vi "Actor Core.vi"(8 "error in":errorcluster, 11 "Alpha UI in":refnum<class "Simulated Entry Console.lvclass">) -> (0 "error out":errorcluster, 3 "Actor out":refnum<class "Actor.lvclass">)   [LabVIEW 2012, in "Simulated Entry Console.lvlib" / "Simulated Entry Console.lvclass"]
doc: "(<B>Filename</B>: Actor Framework.lvlib:Actor.lvclass:Actor Core.vi)\n\nReceives messages to the actor, reacts to them, and initiates any error handling that may shut the actor down.\n\nDescendant classes may override this VI to append parallel tasks for the actor to complete while it handles messages. Overrides use the Call Parent Method node."
uses:
  Simulated Entry Console.lvclass
  <vilib>/ActorFramework/Actor/Actor.lvclass
  <vilib>/ActorFramework/Stop Msg/Stop Msg.lvclass
  Entry Console API/Entry Console API/Entry Console API.lvclass
  Car Wash Controller/Car Wash Controller/Car Wash Controller.lvclass
  Car Wash Controller/Car Wash Controller/Wash Step.ctl
panel:
  in  "Start":bool
  in  "Button 8":bool
  in  "Button 7":bool
  in  "Button 6":bool
  in  "Button 5":bool
  in  "Button 4":bool
  in  "Button 3":bool
  in  "Button 2":bool
  in  "Under Body Wash":bool
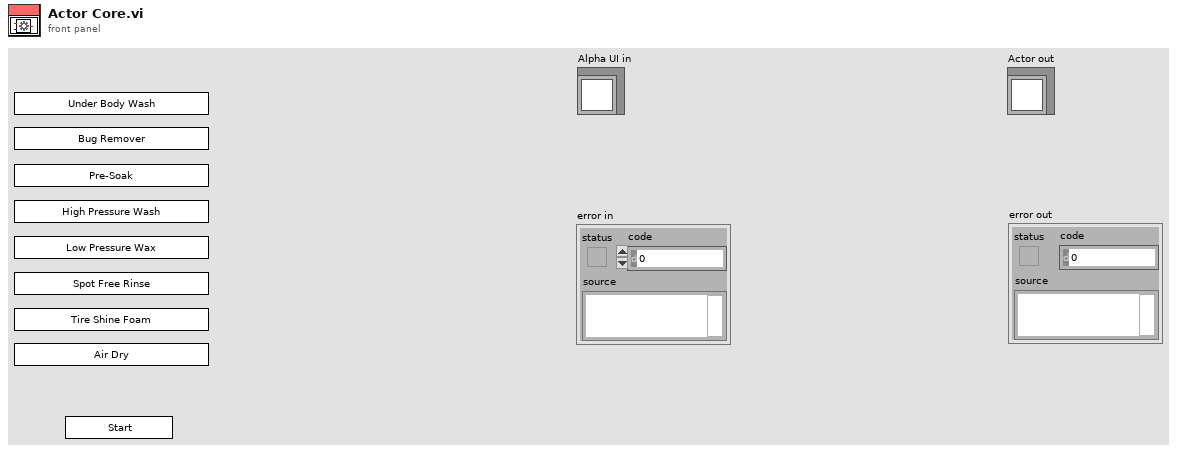
[diagram p1: front panel]
types:
  T1 = typedef "Car Wash Controller.lvlib/Car Wash Controller.lvclass/Wash Step.ctl" = enum16{"Under Body Wash", "Bug Remover", "Pre-Soak", "High Pressure Wash", "Low Pressure Wax", "Spot Free Rince", "Tire Shine Foam", "Air Dry"}
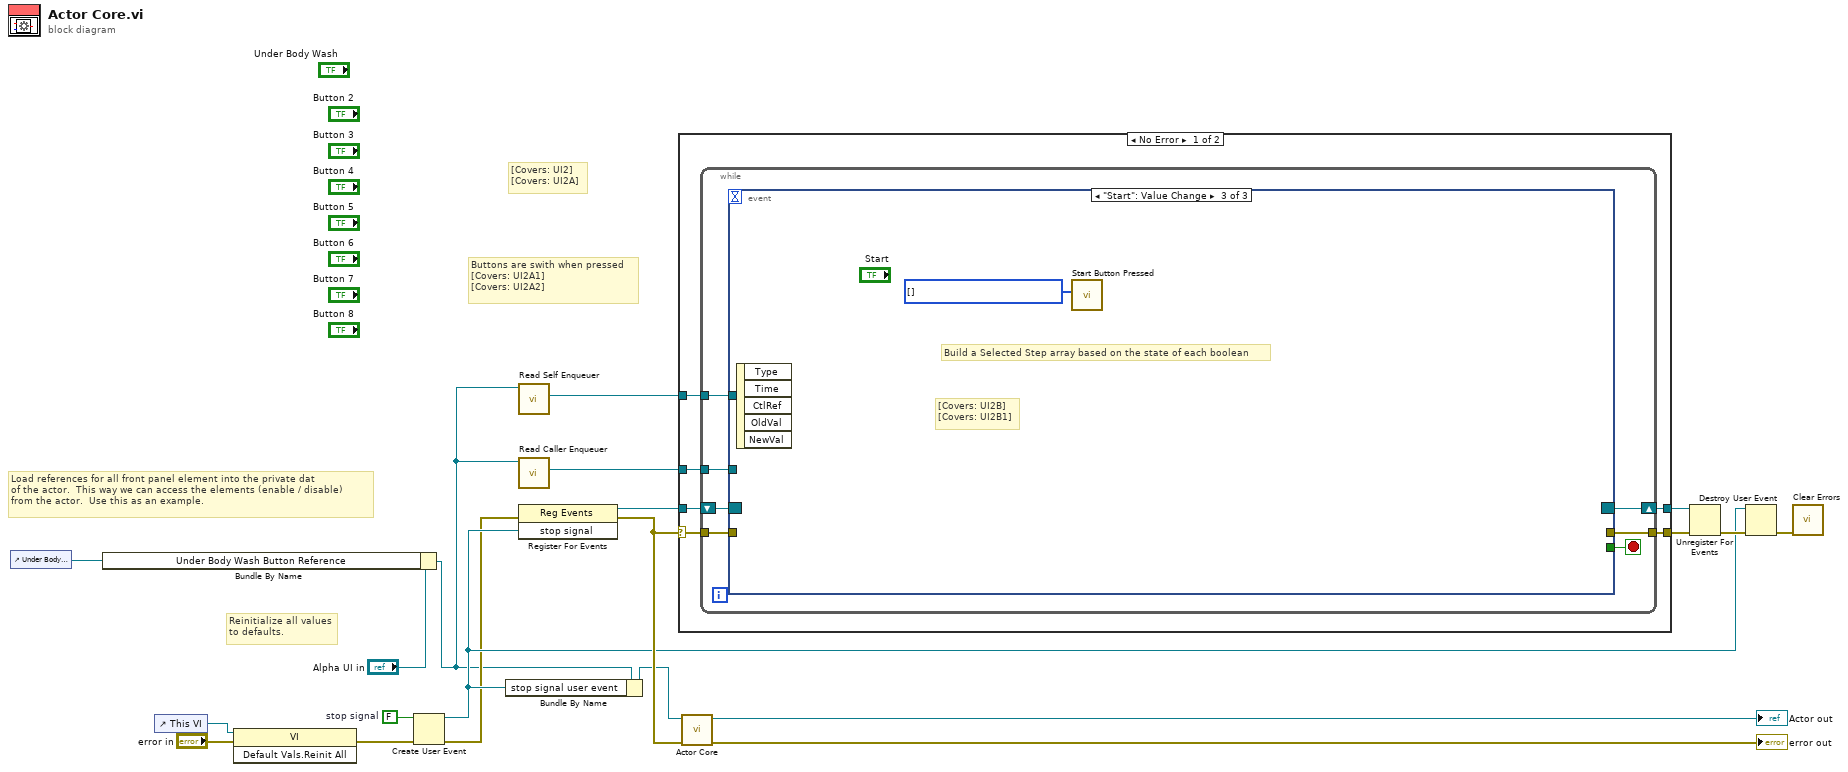
[diagram p0: block diagram]
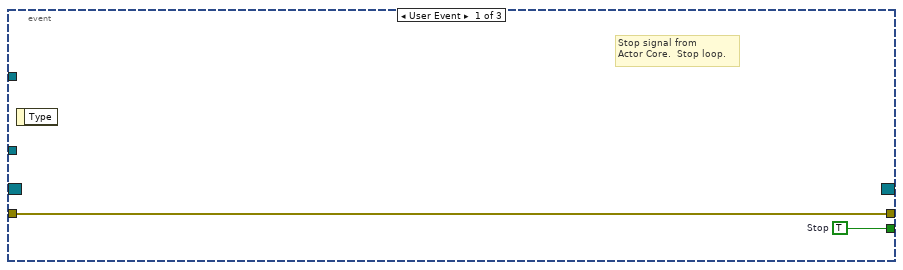
[diagram p2: hidden frame]
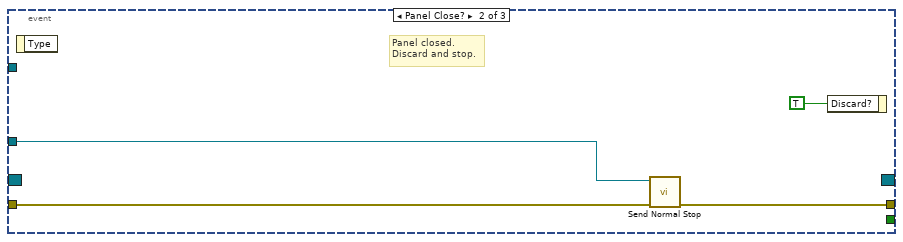
[diagram p3: hidden frame]
diagram:
  w18 = FALSE  # stop signal
  # "Buttons are swith when pressed\n[Covers: UI2A1]\n[Covers: UI2A2]"
  # "[Covers: UI2]\n[Covers: UI2A]"
  # "Load references for all front panel element into the private dat\nof the actor.  This way we can access the elements (enable / disable) \nfrom the actor.  Use this as an example."
  # "Reinitialize all values\nto defaults."
  n1 = control-ref of="Under Body Wash"() -> (w1:refnum<vi>)
  n2 = Bundle By Name(cluster="Alpha UI in", "Under Body Wash Button Reference"=w1) -> (w2:refnum<class "Simulated Entry Console.lvclass">)
  n3 = control-ref of="This VI"() -> (w9:refnum<vi>)
  n4 = invoke class="VI" method="Default Vals.Reinit All"(reference=w9, error in="error in") -> (error out=w7:errorcluster)  [unwired: 1 in, 2 out]
  n5 = Create User Event(user event datatype=w18, error in=w7) -> (user event=w10:refnum<user-event>, error out=w6:errorcluster)
  n6 = Bundle By Name(cluster=w2, "stop signal user event"=w10) -> (w4:refnum<class "Simulated Entry Console.lvclass">)
  n7 = call <vilib>:"Read Self Enqueuer.vi"("Actor"=w2) -> ("Self Enqueuer"=w20:refnum<class "Message Enqueuer.lvclass">)  [unwired: 10 in]
  n8 = call <vilib>:"Read Caller Enqueuer.vi"("Actor"=w2) -> ("Caller Enqueuer"=w19:refnum<class "Message Enqueuer.lvclass">)  [unwired: 10 in]
  n9 = register-events(error in=w6, w10) -> (reference out=w17:refnum<event-registration>, error out=w14:errorcluster)  [unwired: 1 in]
  n10 = case shown="No Error" w14 {
    selector: w14 -> [w21 w41]
    tunnel: w20 -> [w26 _]
    tunnel: w19 -> [w25 _]
    tunnel: w17 -> [w24 w42]
    tunnel: [w23 w42] -> w15
    tunnel: [w22 w41] -> w13
    frame No Error {
      n11 = while {
        tunnel: w26 -> [w32]
        tunnel: w25 -> [w31]
        shift-right: [w29] -> w23
        shift-left: w24 -> [w30]
        tunnel: [w28] -> w22
        tunnel: w21 -> [w27]
        stop <- w33 stop-if-true
        n12 = event shown="[2] \"Start\": Value Change" {
          selector: w30 -> [_ _ _]
          dyn-events: [_ _ _] -> w29
          timeout: _ -> [_ _ _]
          tunnel: [w35 _ _] -> w33
          tunnel: w32 -> [_ _ _]
          tunnel: w31 -> [_ w39 _]
          tunnel: [w34 w38 _] -> w28
          tunnel: w27 -> [w34 w37 _]
          event User Event {
            w35 = TRUE  # Stop
            # "Stop signal from\nActor Core.  Stop loop."
            n13 = event-data() -> ()  [unwired: 1 in, 1 out]
          }
          event Panel Close? {
            # "Panel closed.\nDiscard and stop."
            n14 = event-data() -> ()  [unwired: 1 in, 1 out]
            n15 = call <vilib>:"Send Normal Stop.vi"("error in (no error)"=w37, "Message Enqueuer"=w39) -> ("error out"=w38:errorcluster)  [unwired: 9 in]
            n16 = event-data("Discard?"=TRUE) -> ()  [unwired: 1 in, 1 out]
          }
          event "Start": Value Change {
            w40 = T1[] [] items=["Under Body Wash", "Bug Remover", "Pre-Soak", "High Pressure Wash", "Low Pressure Wax", "Spot Free Rince", "Tire Shine Foam", "Air Dry"] ("Selected Steps")
            # "[Covers: UI2B]\n[Covers: UI2B1]"
            # "Build a Selected Step array based on the state of each boolean"
            n17 = event-data() -> ()  [unwired: 1 in, 5 out]
            n18 = call-dynamic "Start Button Pressed.vi"("Selected Steps"=w40) -> ()  [unwired: 9 in, 2 out]
          }
        }
      }
    }
    frame Error {
    }
  }
  n19 = call-parent "Actor Core.vi"("error in"=w14, "Actor in"=w4) -> ("error out"=→"error out":errorcluster, "Actor out"=→"Actor out":refnum<class "Actor.lvclass">)  [unwired: 8 in]
  n20 = Unregister For Events(event registration refnum=w15, error in=w13) -> (error out=w16:errorcluster)
  n21 = Destroy User Event(user event=w10, error in=w16) -> (error out=w5:errorcluster)
  n22 = call <vilib>:"Clear Errors.vi"("error in (no error)"=w5) -> ()  [unwired: 6 in, 1 out]
